vi "Parse Arguments.vi"(9 "Working Directory":path, 10 "Command Line Args":string[](array[string]), 11 "Parameters in":T1) -> (0 "error constant":errorcluster, 3 "Parameters out":T1)   [LabVIEW 2016]
uses:
  <vilib>/ErrorRing/Error Ring.xnode
  <vilib>/regexp/Match Regular Expression.xnode
  Command Line Arguments.ctl
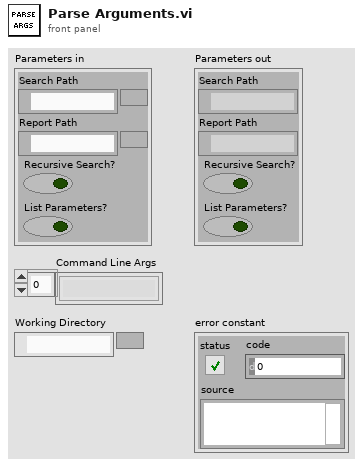
[diagram p1: front panel]
types:
  T1 = typedef "Command Line Arguments.ctl" = cluster{"Search Path":path, "Report Path":path, "Recursive Search?":bool, "List Parameters?":bool}
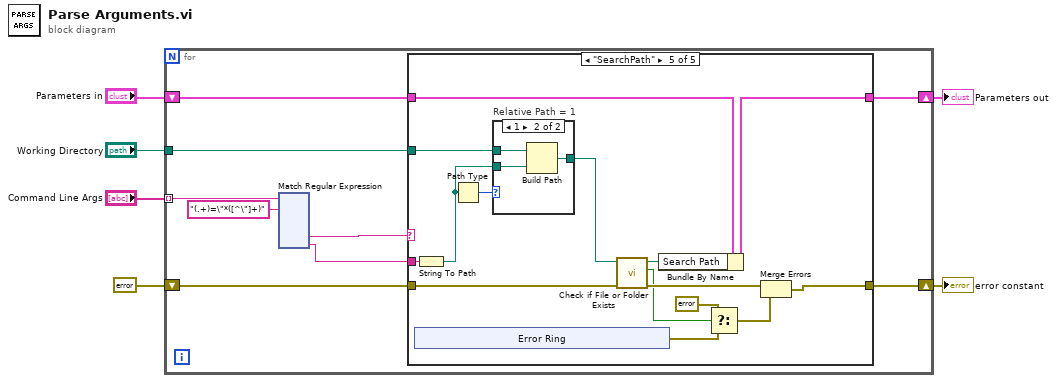
[diagram p0: block diagram]
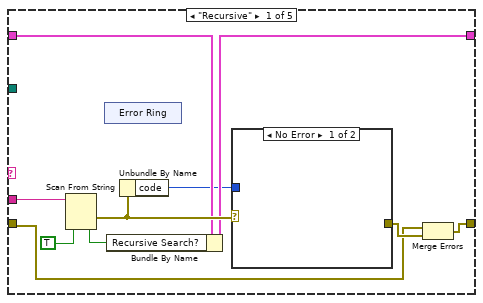
[diagram p2: hidden frame]
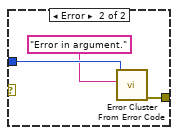
[diagram p3: hidden frame]
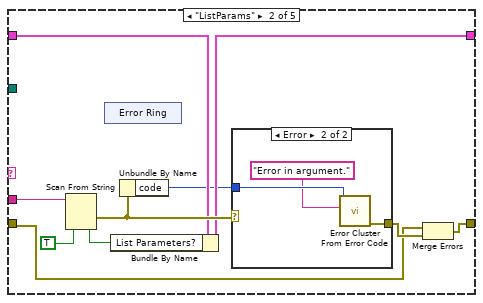
[diagram p4: hidden frame]
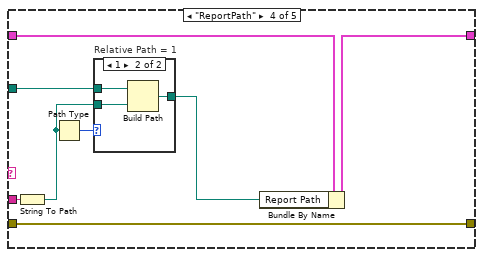
[diagram p7: hidden frame]
diagram:
  n1 = for {
    tunnel: "Command Line Args" -> [w10] mode=indexing
    shift-right: [w12] -> w3
    shift-left: "Parameters in" -> [w13]
    shift-right: [w14] -> w5
    shift-left: errorcluster {"status"=FALSE, "code"=0, "source"=""} ("error constant") -> [w15]
    tunnel: "Working Directory" -> [w7]
    n2 = xnode "Match Regular Expression"("input string"=w10, "regular expression"="(.+)=\"*([^\"]+)") -> ("submatch 1"=w9:string, "submatch 2"=w8:string)  [unwired: 4 in, 5 out]
    n3 = case shown="\"SearchPath\"" w9 {
      tunnel: w8 -> [w137 w151 _ w168 w181]
      tunnel: w13 -> [w138 w152 w161 w170 w183]
      tunnel: [w135 w149 w161 w169 w182] -> w12
      tunnel: w15 -> [w139 w153 w162 w163 w189]
      tunnel: [w140 w154 w162 w163 w187] -> w14
      tunnel: w7 -> [_ _ _ w166 w177]
      frame "Recursive" {
        n4 = Scan From String(input string=w137, default 1=TRUE) -> (error out=w141:errorcluster, output 1=w134:bool)  [unwired: 3 in, 2 out]
        n5 = xnode "Error Ring"() -> ()  [unwired: 1 out]
        n6 = Bundle By Name(cluster=w138, "Recursive Search?"=w134) -> (w135:T1)
        n7 = Unbundle By Name(w141) -> ("code"=w133:i32)
        n8 = case shown="No Error" w141 {
          tunnel: [_ w146] -> w142
          tunnel: w133 -> [_ w145]
          frame No Error {
          }
          frame Error {
            n9 = call <vilib>:"Error Cluster From Error Code.vi"("error message (\"\")"="Error in argument." ("error message (\"\")"), "error code (0)"=w145) -> ("error out"=w146:errorcluster)  [unwired: 7 in]
          }
        }
        n10 = Merge Errors(w139, w142) -> (w140:errorcluster)
      }
      frame "ListParams" {
        n11 = Scan From String(input string=w151, default 1=TRUE) -> (error out=w155:errorcluster, output 1=w148:bool)  [unwired: 3 in, 2 out]
        n12 = xnode "Error Ring"() -> ()  [unwired: 1 out]
        n13 = Bundle By Name(cluster=w152, "List Parameters?"=w148) -> (w149:T1)
        n14 = Unbundle By Name(w155) -> ("code"=w147:i32)
        n15 = case shown="Error" w155 {
          tunnel: [_ w160] -> w156
          tunnel: w147 -> [_ w159]
          frame No Error {
          }
          frame Error {
            n16 = call <vilib>:"Error Cluster From Error Code.vi"("error message (\"\")"="Error in argument." ("error message (\"\")"), "error code (0)"=w159) -> ("error out"=w160:errorcluster)  [unwired: 7 in]
          }
        }
        n17 = Merge Errors(w153, w156) -> (w154:errorcluster)
      }
      frame Default {
      }
      frame "ReportPath" {
        n18 = String To Path(string=w168) -> (path=w165:path)
        n19 = Path Type(1:w165) -> (0:w167:i16)
        n20 = case "Relative Path = 1" shown="1" w167 {
          tunnel: w166 -> [_ w174]
          tunnel: w165 -> [w171 w173]
          tunnel: [w171 w172] -> w164
          frame Default {
          }
          frame 1 {
            n21 = Build Path(base path=w174, name or relative path=w173) -> (appended path=w172:path)
          }
        }
        n22 = Bundle By Name(cluster=w170, "Report Path"=w164) -> (w169:T1)
      }
      frame "SearchPath" {
        n23 = xnode "Error Ring"() -> ("error out"=w186:errorcluster)
        n24 = String To Path(string=w181) -> (path=w176:path)
        n25 = Path Type(1:w176) -> (0:w178:i16)
        n26 = case "Relative Path = 1" shown="1" w178 {
          tunnel: w177 -> [_ w193]
          tunnel: w176 -> [w190 w192]
          tunnel: [w190 w191] -> w175
          frame Default {
          }
          frame 1 {
            n27 = Build Path(base path=w193, name or relative path=w192) -> (appended path=w191:path)
          }
        }
        n28 = call <vilib>:"Check if File or Folder Exists.vi"("error in (no error)"=w189, "path"=w175) -> ("error out"=w188:errorcluster, "file or folder exists?"=w179:bool, "dup path"=w180:path)  [unwired: 7 in]
        n29 = Bundle By Name(cluster=w183, "Search Path"=w180) -> (w182:T1)
        n30 = Select(t=errorcluster {"status"=FALSE, "code"=0, "source"=""} ("error constant"), s=w179, f=w186) -> (s? t:f=w184:errorcluster)
        n31 = Merge Errors(w188, w184) -> (w187:errorcluster)
      }
    }
  }
  "Parameters out" <- w3
  "error constant" <- w5
